vi "Stepper Wait Till Steps Complete.vi"(8 "error in":errorcluster, 11 "Arduino Resource In":T1={"VISA resource"="", "Board Type"=enum."Arduino Uno", "Connection Type"=enum."USB / Serial", "Bytes Per Packet (15)"=15}) -> (0 "error out":errorcluster, 3 "Arduino Resource Out":T1={"VISA resource"="", "Board Type"=enum."Arduino Uno", "Connection Type"=enum."USB / Serial", "Bytes Per Packet (15)"=15})   [LabVIEW 2011, in "LabVIEW Interface for Arduino.lvlib"]
doc: "This VI blocks and allows execution to continue after there are no further stepper commands in need of processing."
uses:
  LabVIEW Interface for Arduino.lvlib
  Private/Type Defs/Arduino Resource.ctl
  Private/Type Defs/Board Type.ctl
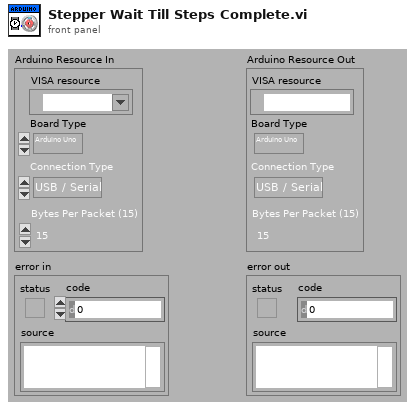
[diagram p1: front panel]
types:
  T1 = typedef "LabVIEW Interface for Arduino.lvlib/Arduino Resource.ctl" = cluster{"VISA resource":refnum<visa-resource-name>, "Board Type":T2, "Connection Type":enum8{"USB / Serial"}, "Bytes Per Packet (15)":u8}
  T2 = typedef "LabVIEW Interface for Arduino.lvlib/Board Type.ctl" = enum16{"Arduino Uno", "Dimuelanove w/Atmega 328", "Mega 2560", "Chipkit Uno32", "Chipkit Max32"}
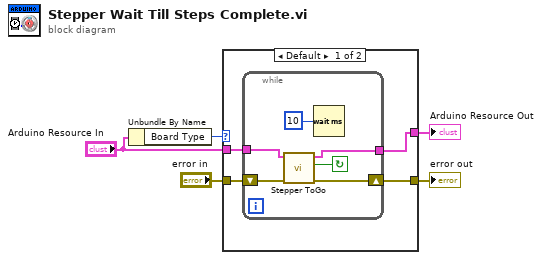
[diagram p0: block diagram]
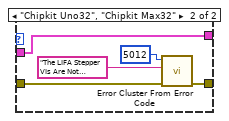
[diagram p2: hidden frame]
diagram:
  n1 = Unbundle By Name("Arduino Resource In") -> ("Board Type"=w4:T2)
  n2 = case shown="Default" w4 {
    tunnel: "Arduino Resource In" -> [w9 w18]
    tunnel: "error in" -> [w8 w16]
    tunnel: [w7 w17] -> w2
    tunnel: [w6 w18] -> w1
    frame Default {
      n3 = while {
        tunnel: [w11] -> w6
        shift-right: [w12] -> w7
        shift-left: w8 -> [w13]
        tunnel: w9 -> [w14]
        stop <- w10 continue-if-true
        n4 = call "Stepper ToGo.vi"("error in"=w13, "Arduino Resource"=w14) -> ("error out"=w12:errorcluster, "Steps Remaining?"=w10:bool, "Arduino Resource Out"=w11:T1)  [unwired: 6 in, 1 out]
        n5 = Wait (ms)(milliseconds to wait=u32 10) -> ()  [unwired: 1 out]
      }
    }
    frame "Chipkit Uno32", "Chipkit Max32" {
      n6 = call <vilib>:"Error Cluster From Error Code.vi"("error in (no error)"=w16, "error message (\"\")"="The LIFA Stepper VIs Are Not Supported On Chipkit Targets." ("source"), "error code (0)"=5012) -> ("error out"=w17:errorcluster)  [unwired: 6 in]
    }
  }
  "error out" <- w2
  "Arduino Resource Out" <- w1
